vi "test_comm.vi"() -> ()   [LabVIEW 2012]
uses:
  CRDS Class/Data Class/Main Class/CRDS Data.lvclass
  CRDS Class/Data Class/Cell Class/CRDS Cell Data.lvclass
  Reusable/CRDS/Data/Main/CRDS Data.lvclass
  Reusable/DataClass/Alicat/MC/AlicatMCData.lvclass
  Reusable/DataClass/TECooler/TECData.lvclass
panel:
  out "current time":timestamp
  out "data string":string
  out "error out":errorcluster
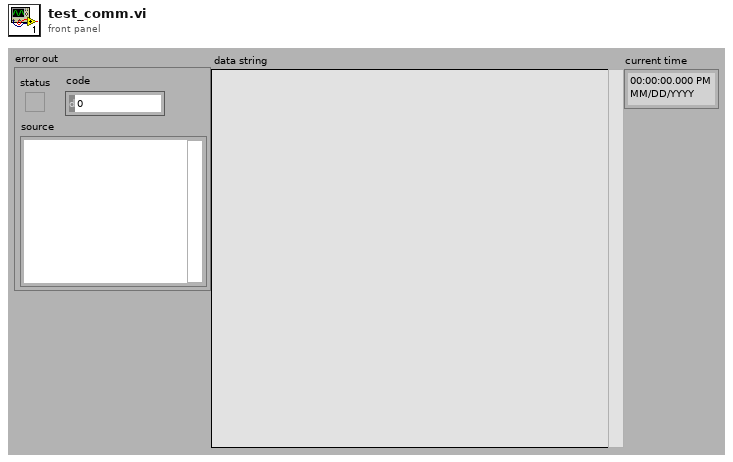
[diagram p1: front panel]
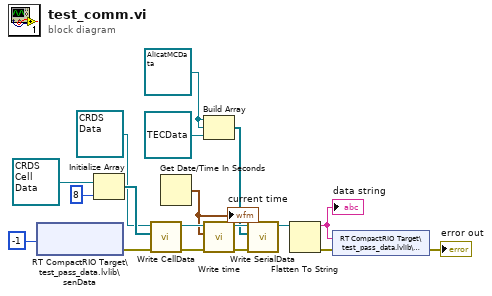
[diagram p0: block diagram]
diagram:
  w4 = refnum<class "AlicatMCData.lvclass"> refnum ("AlicatMCData.lvclass")
  n1 = shared-variable "RT CompactRIO Target\\test_pass_data.lvlib\\senData"(-1 ("ms timeout (0)")) -> (error out=w5:errorcluster)  [unwired: 1 in, 2 out]
  n2 = Initialize Array(refnum<class "CRDS Cell Data.lvclass"> refnum ("CRDS Cell Data.lvclass"), 8 ("dimension size")) -> (w13:refnum<class "CRDS Cell Data.lvclass">[])
  n3 = call "Write CellData.vi"("error in"=w5, "CellData"=w13, "CRDS Data in"=refnum<class "CRDS Data.lvclass"> refnum ("CRDS Data.lvclass")) -> ("error out"=w10:errorcluster, "CRDS Data out"=w11:refnum<class "CRDS Data.lvclass">)  [unwired: 7 in]
  n4 = Get Date/Time In Seconds() -> (seconds since 1Jan1904=w9:timestamp)
  "current time" <- w9
  n5 = Build Array(w4, w4, refnum<class "TECData.lvclass"> refnum ("TECData.lvclass")) -> (w2:refnum<class>[])
  n6 = call "Write time.vi"("error in (no error)"=w10, "time"=w9, "CRDS Data in"=w11) -> ("error out"=w7:errorcluster, "CRDS Data out"=w8:refnum<class "CRDS Data.lvclass">)  [unwired: 7 in]
  n7 = call "Write SerialData.vi"("error in (no error)"=w7, "SerialData"=w2, "CRDS Data in"=w8) -> ("CRDS Data out"=w6:refnum<class "CRDS Data.lvclass">)  [unwired: 7 in, 1 out]
  n8 = Flatten To String(anything=w6) -> (data string=w18:string, error out=w1:errorcluster)  [unwired: 3 in, 1 out]
  "data string" <- w18
  n9 = shared-variable "RT CompactRIO Target\\test_pass_data.lvlib\\CRDdata3"(w18, error in=w1) -> (error out=→"error out":errorcluster)
